vi "AvgWaveform.vi"(2 "error in (no error)":errorcluster, 3 "Waveform Array":waveform(sgl)[](array[waveform])) -> (0 "error out":errorcluster, 1 "Avg waveform":waveform(sgl))   [LabVIEW 2009]
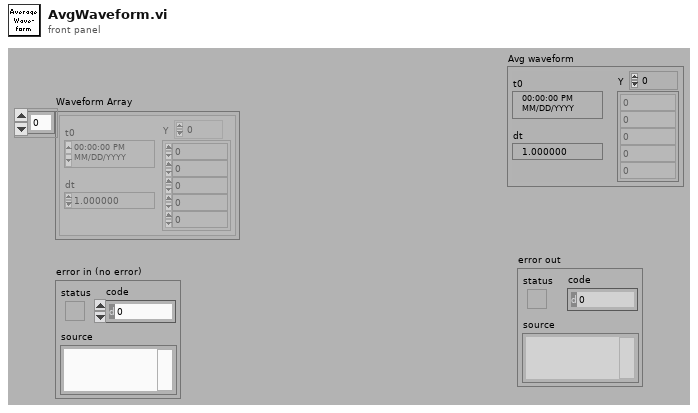
[diagram p1: front panel]
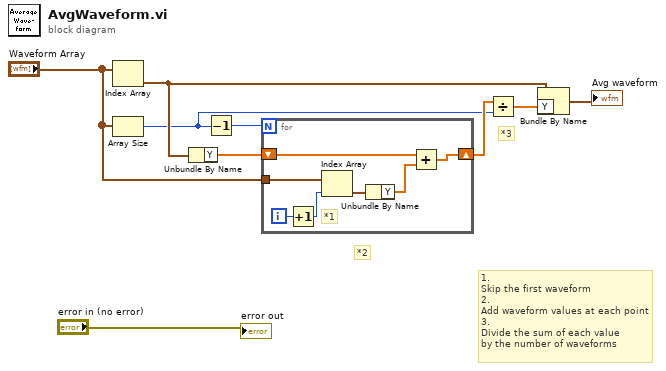
[diagram p0: block diagram]
diagram:
  # "*3"
  # "*2"
  # "1.\nSkip the first waveform\n2.\nAdd waveform values at each point\n3.\nDivide the sum of each value\nby the number of waveforms"
  n1 = Index Array(array="Waveform Array") -> (element=w7:waveform(sgl))  [unwired: 1 in]
  n2 = Array Size(array="Waveform Array") -> (size(s)=w3:i32)
  n3 = Unbundle By Name(w7) -> ("Y"=w4:sgl[])
  n4 = Decrement(x=w3) -> (x-1=w2:i32)
  n5 = for {
    N: w2 -> [_]
    tunnel: "Waveform Array" -> [w13]
    shift-right: [w14] -> w9
    shift-left: w4 -> [w15]
    i -> [w11]
    # "*1"
    n6 = Increment(x=w11) -> (x+1=w10:i32)
    n7 = Index Array(array=w13, index=w10) -> (element=w12:waveform(sgl))
    n8 = Unbundle By Name(w12) -> ("Y"=w16:sgl[])
    n9 = Add(x=w15, y=w16) -> (x+y=w14:sgl[])
  }
  n10 = Divide(x=w9, y=w3) -> (x/y=w8:sgl[])
  n11 = Bundle By Name(cluster=w7, "Y"=w8) -> (→"Avg waveform":waveform(sgl))
  "error out" <- "error in (no error)"
